vi "Get VI Path for Response Message.vi"(8 "error in (no error)":errorcluster, 11 "Process Ptah":path) -> (0 "error out":errorcluster, 3 "Path":path)   [LabVIEW 2020, in "Method Generation.lvlib" / "Getter Generator.lvclass"]
uses:
  Getter Generator.lvclass
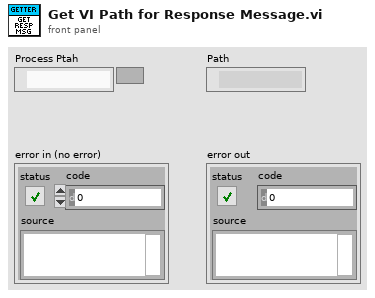
[diagram p1: front panel]
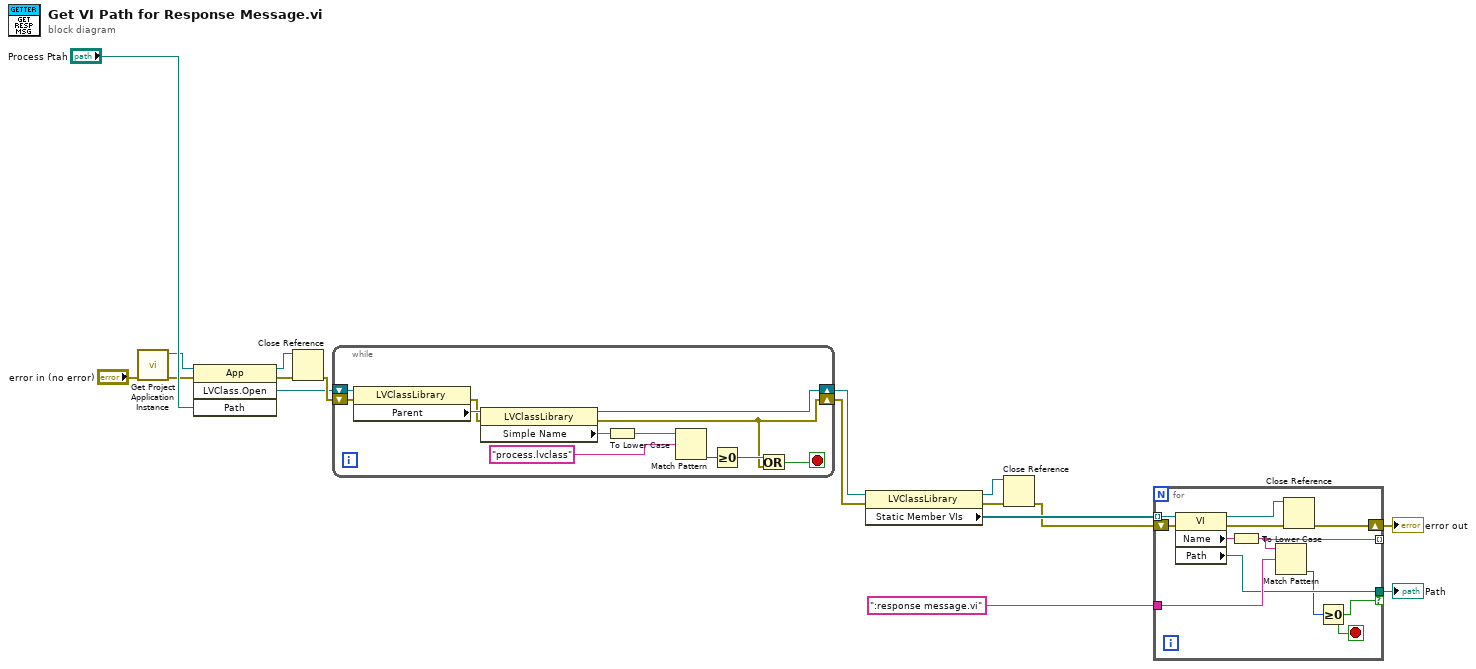
[diagram p0: block diagram]
diagram:
  n1 = call "Get Project Application Instance.vi"("error in (no error)"="error in (no error)") -> ("error out"=w6:errorcluster, "Application out"=w5:refnum<vi>)  [unwired: 9 in]
  n2 = invoke class="App" method="LVClass.Open"(reference=w5, error in=w6, "Path"="Process Ptah") -> (reference out=w8:refnum<vi>, error out=w7:errorcluster, "LVClass.Open"=w14:refnum<vi>)  [unwired: 1 in, 1 out]
  n3 = Close Reference(reference=w8, error in (no error)=w7) -> (error out=w15:errorcluster)
  n4 = while {
    shift-right: [w27] -> w16
    shift-left: w14 -> [w29]
    shift-right: [w18] -> w3
    shift-left: w15 -> [w25]
    stop <- w19 stop-if-true
    n5 = property class="LVClassLibrary"(reference=w29, error in=w25) -> (error out=w26:errorcluster, "Parent"=w28:refnum<vi>)  [unwired: 1 out]
    n6 = property class="LVClassLibrary"(reference=w28, error in=w26) -> (reference out=w27:refnum<vi>, error out=w18:errorcluster, "Simple Name"=w24:string)
    n7 = To Lower Case(string=w24) -> (all lower case string=w23:string)
    n8 = Match Pattern(string=w23, regular expression="process.lvclass") -> (offset past match=w20:i32)  [unwired: 1 in, 3 out]
    n9 = Greater Or Equal To 0?(x=w20) -> (x >= 0?=w21:bool)
    n10 = Or(x=w21, y=w18) -> (x .or. y?=w19:bool)
  }
  n11 = property class="LVClassLibrary"(reference=w16, error in=w3) -> (reference out=w13:refnum<vi>, error out=w12:errorcluster, "Static Member VIs"=w10:refnum<vi>[])
  n12 = Close Reference(reference=w13, error in (no error)=w12) -> (error out=w2:errorcluster)
  n13 = for {
    tunnel: w10 -> [w40] mode=indexing
    tunnel: ":response message.vi" -> [w39]
    tunnel: [w38] -> w17 if=w32
    tunnel: [w33] -> _ mode=indexing
    shift-right: [w30] -> w1
    shift-left: w2 -> [w31]
    stop <- w32 stop-if-true
    n14 = property class="VI"(reference=w40, error in=w31) -> (reference out=w36:refnum<vi>, error out=w37:errorcluster, "Name"=w35:string, "Path"=w38:path)
    n15 = To Lower Case(string=w35) -> (all lower case string=w33:string)
    n16 = Match Pattern(string=w33, regular expression=w39) -> (offset past match=w34:i32)  [unwired: 1 in, 3 out]
    n17 = Close Reference(reference=w36, error in (no error)=w37) -> (error out=w30:errorcluster)
    n18 = Greater Or Equal To 0?(x=w34) -> (x >= 0?=w32:bool)
  }
  "Path" <- w17
  "error out" <- w1
